vi "TDC_setTimestampBufferSize.vi"(8 "Error In":errorcluster, 11 "Buffer Size":i32 min=1 max=1000000) -> (0 "Error Out":errorcluster)   [LabVIEW 2011]
uses:
  tdcbase.dll
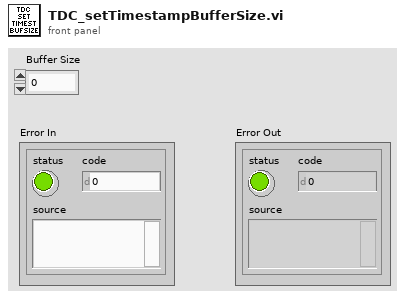
[diagram p1: front panel]
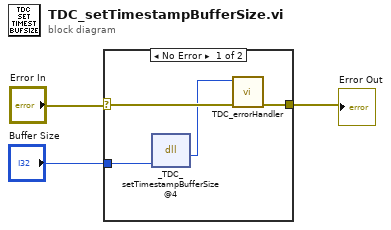
[diagram p0: block diagram]
diagram:
  n1 = case shown="No Error" "Error In" {
    selector: "Error In" -> [w6 w8]
    tunnel: [w5 w8] -> w3
    tunnel: "Buffer Size" -> [w7 _]
    frame No Error {
      n2 = dll-call lib="X:/tdcbase.dll" fn="_TDC_setTimestampBufferSize@4"("bufferSize"=w7) -> ("return type"=w4:i32)  [unwired: 4 in, 2 out]
      n3 = call "TDC_errorHandler.vi"("Error In"=w6, "TDC Return Code"=w4) -> ("Error Out"=w5:errorcluster)  [unwired: 9 in]
    }
    frame Error {
    }
  }
  "Error Out" <- w3
